vi "realtime_IV_K2182A_K6221_vs_time_PK.vi"() -> ()   [LabVIEW 2016]
uses:
  Labview Drivers/Keithley 622x LV 2009/Keithley 622x LV 2009/Utility/Typedefs/KE622x -- Instrument Type.ctl
  \\home2\scratch/Heng/Vread vs time program/C/Program Files/National Instruments/LabVIEW 2016/instr.lib/Keithley 2182/Keithley 2182.lvlib
  Labview Drivers/Keithley 622x LV 2009/Keithley 622x.lvlib
panel:
  in  "Compliance Voltage (V)":dbl=2.0 format="%#_13g"
  in  "Measurement time (s)":i32=5
  in  "I low (A)":dbl=3.5e-05 format="%#_13g"
  in  "I high (A)":dbl=3.5e-05 format="%#_13g"
  in  "milliseconds to wait":u32=50
  out "Current (A)":dbl=3.5e-05
  out "Voltage, Current vs time":cluster{dbl[], dbl[]}[](graph)=[{[0.09001120005268604, 0.17392860003747046, 0.25689580000471324, 0.34132849995512515, 0.42540299997199327, 0.5330105000175536, 0.616786599974148, 0.7007576000178233, 0.7859523999504745, 0.8734561000019312, 0.9573167000198737, 1.0410527000203729, 1.123987799976021, 1.2319731999887154, 1.3157297000288963, 1.3994928000029176, 1.4842683000024408, 1.567963800043799, 1.6757461000233889, 1.7604933000402525, 1.8453336999518797, 1.9281911000143737, 2.011828999966383, 2.1194837000221014, 2.2033508999738842, 2.288044400047511, 2.3720796999987215, 2.455827399971895, 2.564476400031708, 2.648404399980791, 2.732585599995218, 2.8160608999896795, 2.899973400053568, 3.0093368999660015, 3.0932457000017166, 3.1782505000010133, 3.2620929999975488, 3.34611279994715, 3.4536611000075936, 3.53644890000578, 3.619862799998373, 3.7043840000405908, 3.787445200025104, 3.8964777999790385, 3.9805380000034347, 4.06360069999937, 4.147366099990904, 4.2313554000575095, 4.342785699991509, 4.42666899994947, 4.510417400044389, 4.594143499969505, 4.677875300054438, 4.7866037000203505, 4.868433300056495, 4.950147600029595, 5.03403740003705, 5.116245900047943, 5.225699799950235, 5.309295200044289, 5.392163599957712, 5.475838299957104, 5.559273199993186, 5.668193200021051, 5.751985499984585, 5.8357585000339895, 5.92049509997014, 6.004160400014371, 6.112092899973504, 6.195801900001243, 6.2805609999923036, 6.364234099979512, 6.448114800034091, 6.556113400030881, 6.639614199986681, 6.723240699968301, 6.807079700054601, 6.891112699988298, 6.999815399991348, 7.0835898000514135, 7.167793800006621, 7.251457900041714, 7.335164400050417, 7.442889400059357, 7.525731400004588, 7.609408600023016, 7.693278899998404, 7.776963599957526, 7.887556300032884, 7.971557899960317, 8.055263599962927, 8.139243199955672, 8.221872400026768, 8.376425900030881, 8.460303799947724, 8.544166299980134, 8.627897000056691, 8.711752300034277, 8.819434399949387, 8.902712399954908, 8.985357800032943, 9.069069199962541, 9.152736100018956, 9.261347300023772, 9.344197700032964, 9.4280402000295, 9.512762399972416, 9.59685970004648, 9.707502600038424, 9.789378299959935, 9.873171100043692, 9.956881299964152, 10.040252799983136, 10.149399799993262, 10.232639400055632, 10.315507599967532, 10.39811239996925, 10.483006999944337, 10.589900000020862, 10.673453800030984, 10.75625510001555, 10.838458999991417, 10.921870499965735, 11.030491200042889, 11.112396799959242, 11.195403899997473, 11.279033600003459, 11.36295560002327, 11.47256689995993, 11.556370600010268, 11.639203600003384, 11.723033200018108, 11.806714799953625, 11.915487900027074, 11.997212399961427, 12.081089899991639, 12.164966500014998, 12.248737000045367, 12.357347400044091, 12.439515799982473, 12.523037999984808, 12.606748000020161, 12.69069269997999, 12.798886899952777, 12.882544600055553, 12.966471399995498, 13.050215000053868, 13.134237400023267, 13.245849599945359, 13.329620899981819, 13.413423900026828, 13.497106299968436, 13.580901199951768, 13.688763599959202, 13.772477800026536, 13.856217900058255, 13.939937900053337, 14.02286400005687, 14.131848799996078, 14.215486999950372, 14.299411899992265, 14.383130199974403, 14.466931400005706, 14.574997700052336, 14.658611900056712], [2.01901868e-05, 3.5e-05, 2.02808084e-05, 3.5e-05, 2.01789231e-05, 3.5e-05, 2.01968426e-05, 3.5e-05, 2.0146668e-05, 3.5e-05, 2.02485533e-05, 3.5e-05, 2.02813204e-05, 3.5e-05, 2.01953067e-05, 3.5e-05, 2.02132262e-05, 3.5e-05, 2.0222954e-05, 3.5e-05, 2.00949573e-05, 3.5e-05, 2.01691954e-05, 3.5e-05, 2.02055464e-05, 3.5e-05, 2.01482039e-05, 3.5e-05, 2.02342177e-05, 3.5e-05, 2.01973546e-05, 3.5e-05, 2.02531612e-05, 3.5e-05, 2.01968426e-05, 3.5e-05, 2.02649368e-05, 3.5e-05, 2.01610036e-05, 3.5e-05, 2.02690327e-05, 3.5e-05, 2.01338683e-05, 3.5e-05, 2.02654488e-05, 3.5e-05, 2.01901868e-05, 3.5e-05, 2.02342281e-05, 3.5e-05, 2.02122127e-05, 3.5e-05, 2.01912213e-05, 3.5e-05, 2.01942932e-05, 3.5e-05, 2.02178446e-05, 3.5e-05, 2.01702298e-05, 3.5e-05, 2.01548702e-05, 3.5e-05, 2.02250124e-05, 3.5e-05, 2.01558942e-05, 3.5e-05, 2.02577795e-05, 3.5e-05, 2.01784216e-05, 3.5e-05, 2.02219405e-05, 3.5e-05, 2.02050449e-05, 3.5e-05, 2.02127247e-05, 3.5e-05, 2.02132367e-05, 3.5e-05, 2.0200437e-05, 3.5e-05, 2.01405346e-05, 3.5e-05, 2.01328548e-05, 3.5e-05, 2.02096528e-05, 3.5e-05, 2.01302948e-05, 3.5e-05, 2.01364387e-05, 3.5e-05, 2.01512863e-05, 3.5e-05, 2.02931066e-05, 3.5e-05, 2.01773976e-05, 3.5e-05, 2.02265483e-05, 3.5e-05, 2.01594781e-05, 3.5e-05, 2.02311562e-05, 3.5e-05, 2.0124151e-05, 3.5e-05, 2.02434439e-05, 3.5e-05, 2.01497503e-05, 3.5e-05, 2.02229644e-05, 3.5e-05, 2.01523103e-05, 3.5e-05, 2.01948052e-05, 3.5e-05, 2.0125687e-05, 3.5e-05, 2.0163062e-05, 3.5e-05, 2.01932692e-05, 3.5e-05, 2.00929198e-05, 3.5e-05, 2.02285963e-05, 3.5e-05, 2.01389986e-05, 3.5e-05, 2.02055569e-05, 3.5e-05, 2.01277349e-05, 3.5e-05, 2.01799575e-05, 3.5e-05, 2.01942932e-05, 3.5e-05, 2.01533342e-05, 3.5e-05, 2.0200949e-05, 3.5e-05, 2.01026476e-05, 3.5e-05, 2.01809815e-05, 3.5e-05, 2.00898479e-05, 3.5e-05, 2.01656219e-05, 3.5e-05, 2.01364387e-05, 3.5e-05, 2.01968572e-05, 3.5e-05, 2.008934e-05, 3.5e-05, 2.01226191e-05, 3.5e-05, 2.01144273e-05, 3.5e-05, 2.01077715e-05, 3.5e-05, 2.01128914e-05, 3.5e-05, 2.01057235e-05, 3.5e-05, 2.01799616e-05, 3.5e-05, 2.01748418e-05]}, {[0.09001120005268604, 0.17392860003747046, 0.25689580000471324, 0.34132849995512515, 0.42540299997199327, 0.5330105000175536, 0.616786599974148, 0.7007576000178233, 0.7859523999504745, 0.8734561000019312, 0.9573167000198737, 1.0410527000203729, 1.123987799976021, 1.2319731999887154, 1.3157297000288963, 1.3994928000029176, 1.4842683000024408, 1.567963800043799, 1.6757461000233889, 1.7604933000402525, 1.8453336999518797, 1.9281911000143737, 2.011828999966383, 2.1194837000221014, 2.2033508999738842, 2.288044400047511, 2.3720796999987215, 2.455827399971895, 2.564476400031708, 2.648404399980791, 2.732585599995218, 2.8160608999896795, 2.899973400053568, 3.0093368999660015, 3.0932457000017166, 3.1782505000010133, 3.2620929999975488, 3.34611279994715, 3.4536611000075936, 3.53644890000578, 3.619862799998373, 3.7043840000405908, 3.787445200025104, 3.8964777999790385, 3.9805380000034347, 4.06360069999937, 4.147366099990904, 4.2313554000575095, 4.342785699991509, 4.42666899994947, 4.510417400044389, 4.594143499969505, 4.677875300054438, 4.7866037000203505, 4.868433300056495, 4.950147600029595, 5.03403740003705, 5.116245900047943, 5.225699799950235, 5.309295200044289, 5.392163599957712, 5.475838299957104, 5.559273199993186, 5.668193200021051, 5.751985499984585, 5.8357585000339895, 5.92049509997014, 6.004160400014371, 6.112092899973504, 6.195801900001243, 6.2805609999923036, 6.364234099979512, 6.448114800034091, 6.556113400030881, 6.639614199986681, 6.723240699968301, 6.807079700054601, 6.891112699988298, 6.999815399991348, 7.0835898000514135, 7.167793800006621, 7.251457900041714, 7.335164400050417, 7.442889400059357, 7.525731400004588, 7.609408600023016, 7.693278899998404, 7.776963599957526, 7.887556300032884, 7.971557899960317, 8.055263599962927, 8.139243199955672, 8.221872400026768, 8.376425900030881, 8.460303799947724, 8.544166299980134, 8.627897000056691, 8.711752300034277, 8.819434399949387, 8.902712399954908, 8.985357800032943, 9.069069199962541, 9.152736100018956, 9.261347300023772, 9.344197700032964, 9.4280402000295, 9.512762399972416, 9.59685970004648, 9.707502600038424, 9.789378299959935, 9.873171100043692, 9.956881299964152, 10.040252799983136, 10.149399799993262, 10.232639400055632, 10.315507599967532, 10.39811239996925, 10.483006999944337, 10.589900000020862, 10.673453800030984, 10.75625510001555, 10.838458999991417, 10.921870499965735, 11.030491200042889, 11.112396799959242, 11.195403899997473, 11.279033600003459, 11.36295560002327, 11.47256689995993, 11.556370600010268, 11.639203600003384, 11.723033200018108, 11.806714799953625, 11.915487900027074, 11.997212399961427, 12.081089899991639, 12.164966500014998, 12.248737000045367, 12.357347400044091, 12.439515799982473, 12.523037999984808, 12.606748000020161, 12.69069269997999, 12.798886899952777, 12.882544600055553, 12.966471399995498, 13.050215000053868, 13.134237400023267, 13.245849599945359, 13.329620899981819, 13.413423900026828, 13.497106299968436, 13.580901199951768, 13.688763599959202, 13.772477800026536, 13.856217900058255, 13.939937900053337, 14.02286400005687, 14.131848799996078, 14.215486999950372, 14.299411899992265, 14.383130199974403, 14.466931400005706, 14.574997700052336, 14.658611900056712], [3.5e-05, 2.01727793e-05, 3.5e-05, 2.02393375e-05, 3.5e-05, 2.02132262e-05, 3.5e-05, 2.02552091e-05, 3.5e-05, 2.02024745e-05, 3.5e-05, 2.02255139e-05, 3.5e-05, 2.01502519e-05, 3.5e-05, 2.02475293e-05, 3.5e-05, 2.01220926e-05, 3.5e-05, 2.02347296e-05, 3.5e-05, 2.01615156e-05, 3.5e-05, 2.02552091e-05, 3.5e-05, 2.02086183e-05, 3.5e-05, 2.01953067e-05, 3.5e-05, 2.01226046e-05, 3.5e-05, 2.02695447e-05, 3.5e-05, 2.01569077e-05, 3.5e-05, 2.02188581e-05, 3.5e-05, 2.0183019e-05, 3.5e-05, 2.01947947e-05, 3.5e-05, 2.01748272e-05, 3.5e-05, 2.02101543e-05, 3.5e-05, 2.01666354e-05, 3.5e-05, 2.01558942e-05, 3.5e-05, 2.01861014e-05, 3.5e-05, 2.02070928e-05, 3.5e-05, 2.01820055e-05, 3.5e-05, 2.01779096e-05, 3.5e-05, 2.02280843e-05, 3.5e-05, 2.01661339e-05, 3.5e-05, 2.02183566e-05, 3.5e-05, 2.01912213e-05, 3.5e-05, 2.01809815e-05, 3.5e-05, 2.02296203e-05, 3.5e-05, 2.01517983e-05, 3.5e-05, 2.02613634e-05, 3.5e-05, 2.02495877e-05, 3.5e-05, 2.0240372e-05, 3.5e-05, 2.01364387e-05, 3.5e-05, 2.02070928e-05, 3.5e-05, 2.02035089e-05, 3.5e-05, 2.02229644e-05, 3.5e-05, 2.01799575e-05, 3.5e-05, 2.01922452e-05, 3.5e-05, 2.02035089e-05, 3.5e-05, 2.02157966e-05, 3.5e-05, 2.01804695e-05, 3.5e-05, 2.01973651e-05, 3.5e-05, 2.01072554e-05, 3.5e-05, 2.02117007e-05, 3.5e-05, 2.02137487e-05, 3.5e-05, 2.02050449e-05, 3.5e-05, 2.02367881e-05, 3.5e-05, 2.01881493e-05, 3.5e-05, 2.0199413e-05, 3.5e-05, 2.01948052e-05, 3.5e-05, 2.01692058e-05, 3.5e-05, 2.01768856e-05, 3.5e-05, 2.0238324e-05, 3.5e-05, 2.01507743e-05, 3.5e-05, 2.01425825e-05, 3.5e-05, 2.01712538e-05, 3.5e-05, 2.01471904e-05, 3.5e-05, 2.01814935e-05, 3.5e-05, 2.01400226e-05, 3.5e-05, 2.02183566e-05, 3.5e-05, 2.01441185e-05, 3.5e-05, 2.02219405e-05, 3.5e-05, 2.01748377e-05, 3.5e-05, 2.01477024e-05, 3.5e-05, 2.01912213e-05, 3.5e-05, 2.01420705e-05, 3.5e-05, 2.0201973e-05, 3.5e-05, 2.00918999e-05, 3.5e-05, 2.0203001e-05, 3.5e-05, 2.0087804e-05, 3.5e-05, 2.01850815e-05, 3.5e-05, 2.01046996e-05, 3.5e-05, 2.0128763e-05, 3.5e-05, 2.00688605e-05, 3.5e-05, 2.01789377e-05, 3.5e-05, 2.00791002e-05, 3.5e-05]}]
  in  "Instrument Type":T1=enum."KE6221"
  in  "K6221":refnum<visa-resource-name>="GPIB0::12::INSTR"
  out "Time(s)":dbl=14.742446399992332 format="%#_13g"
  in  "?":bool
  out "Voltage (V)":dbl=2.01748418e-05
  in  "Folder":path=path "D:/Banabir/Second round/11-04-2021"
  out "data":dbl[](array[numeric])=[14.658611900056712, 3.5e-05, 2.01748418e-05]
  in  "Nanovoltmeter K2182A VISA (Device 1)":refnum<visa-resource-name>="GPIB0::4::INSTR"
  in  "file name":string="test6"
  out "File path":path=path "D:/Banabir/Second round/11-04-2021/test6.dat"
  # ".dat"
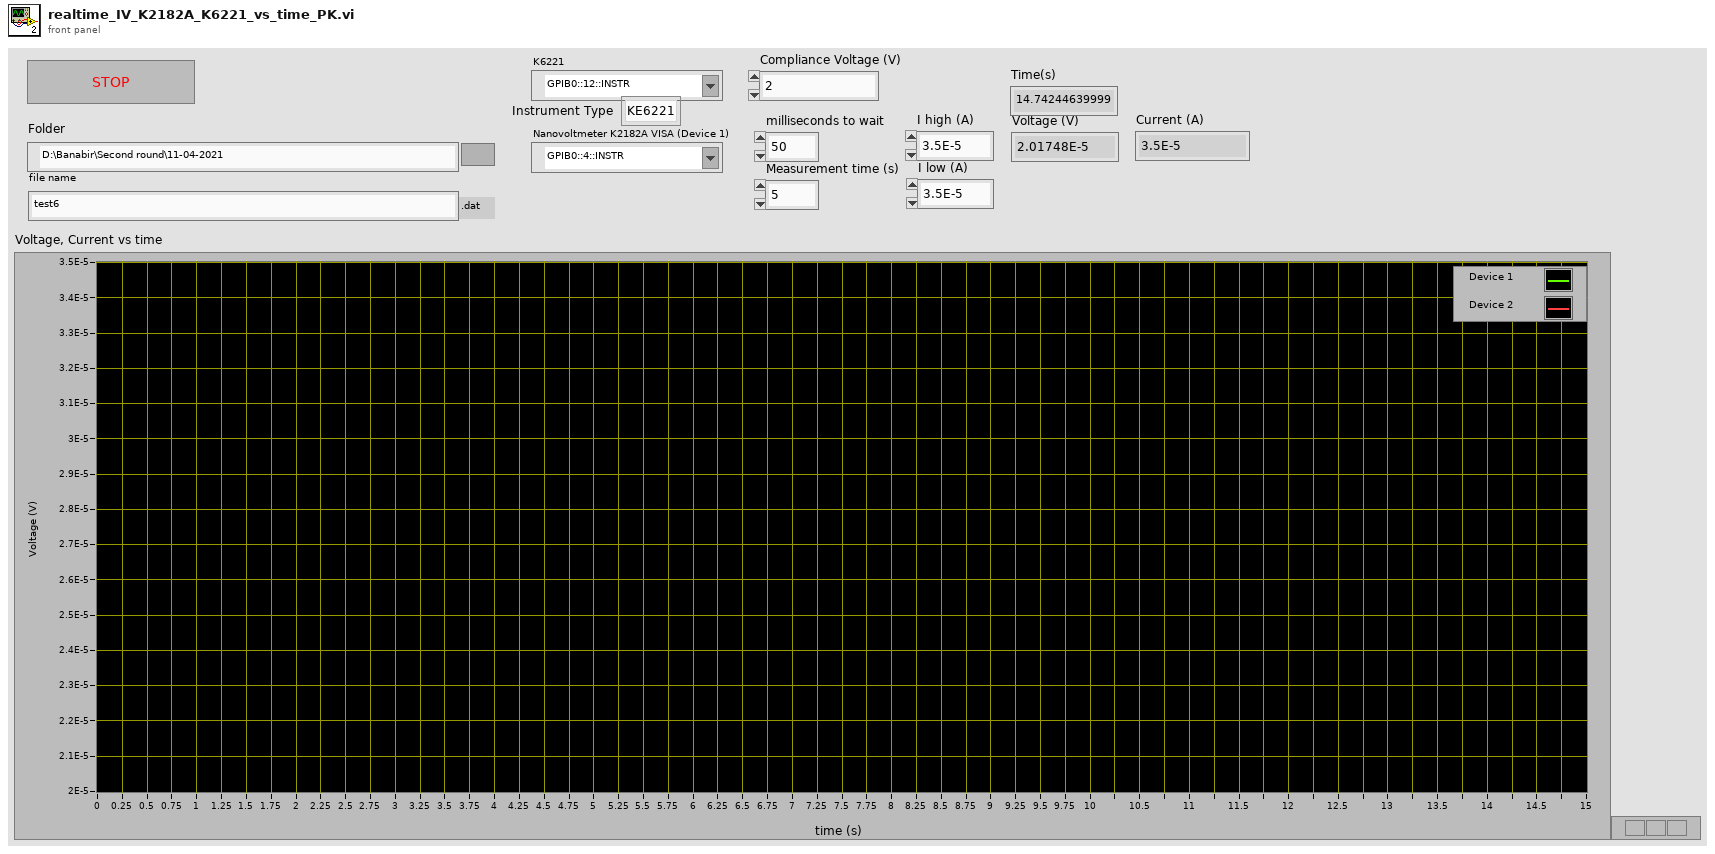
[diagram p1: front panel]
types:
  T1 = typedef "Keithley 622x.lvlib/KE622x -- Instrument Type.ctl" = enum16{"KE6220", "KE6221"}
  T2 = enum16{"open", "replace", "create", "open or create", "replace or create", "replace or create with confirmation"}
  T3 = typedef "Keithley 622x.lvlib/KE622x -- Current Level.ctl" = dbl
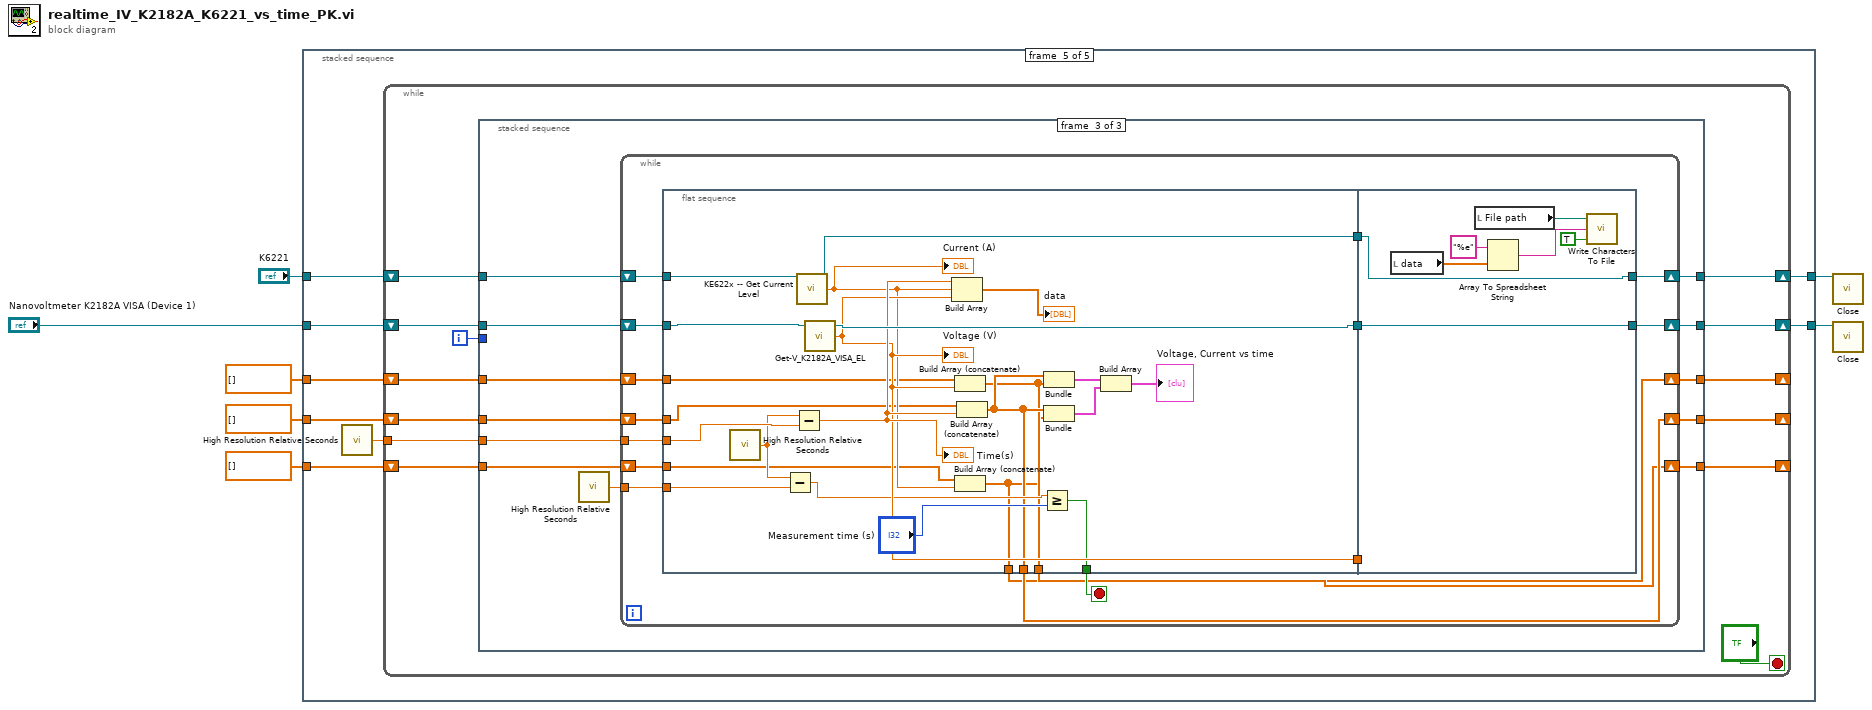
[diagram p0: block diagram]
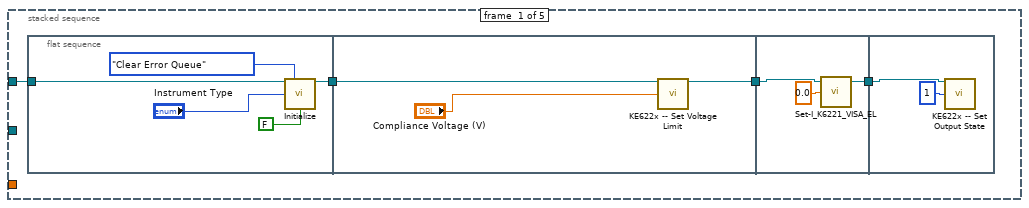
[diagram p2: hidden frame]
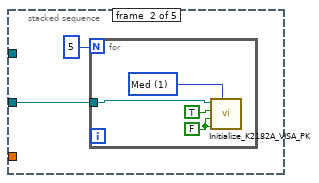
[diagram p3: hidden frame]
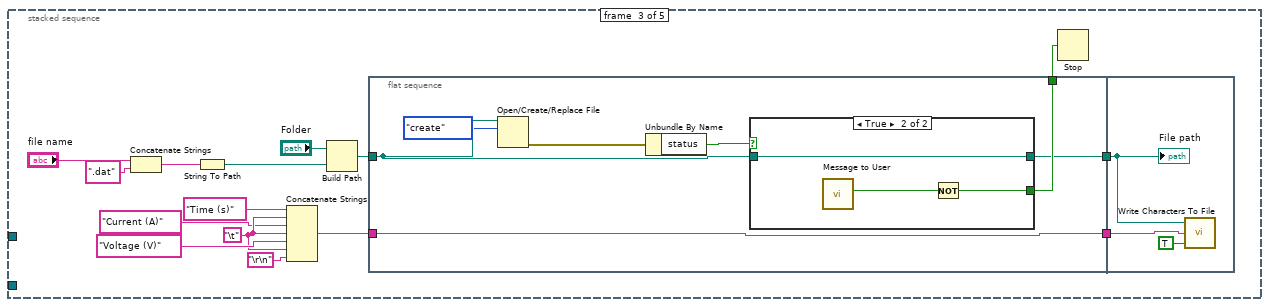
[diagram p4: hidden frame]
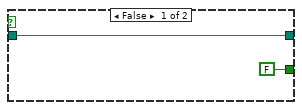
[diagram p5: hidden frame]
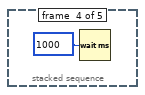
[diagram p6: hidden frame]
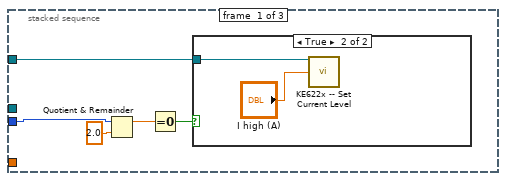
[diagram p7: hidden frame]
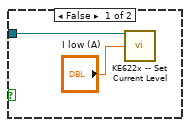
[diagram p8: hidden frame]
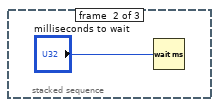
[diagram p9: hidden frame]
diagram:
  n1 = stacked-sequence {
    tunnel: "Nanovoltmeter K2182A VISA (Device 1)" -> [_ w25 _ _ w69]
    tunnel: [_ _ _ _ w67] -> w6
    tunnel: "K6221" -> [w11 _ _ _ w66]
    tunnel: [_ _ _ _ w65] -> w4
    tunnel: dbl[] [] -> [_ _ _ _ w64]
    tunnel: dbl[] [] -> [_ _ _ _ w63]
    tunnel: dbl[] [] -> [_ _ _ _ w62]
    frame #0 {
      n2 = flat-sequence {
        tunnel: w11 -> [w16]
        tunnel: [w15] -> w9
        tunnel: w9 -> [w18]
        tunnel: [w19] -> w8
        tunnel: w8 -> [w21]
        tunnel: [w20] -> w10
        tunnel: w10 -> [w23]
        frame #0 {
          n3 = call "Initialize.vi"("VISA resource name"=w16, "Error Queue Option"=enum16{"Clear Error Queue", "Error Query"}."Clear Error Queue", "Instrument Type"="Instrument Type", "Reset? (T)"=FALSE) -> ("VISA resource name out"=w15:refnum<visa-resource-name>)  [unwired: 10 in, 1 out]
        }
        frame #1 {
          n4 = call "KE622x -- Set Voltage Limit.vi"("Resource In"=w18, "Voltage Limit (V)"="Compliance Voltage (V)") -> ("Resource Out (dupl)"=w19:refnum<visa-resource-name>)  [unwired: 12 in, 1 out]
        }
        frame #2 {
          n5 = call "Set-I_K6221_VISA_EL.vi"("Set I (A)"=0.0, "K6221 VISA"=w21) -> ("K6221 VISA out"=w20:refnum<visa-resource-name>)  [unwired: 2 in, 1 out]
        }
        frame #3 {
          n6 = call "KE622x -- Set Output State.vi"("Resource In"=w23, "Output State"=1) -> ()  [unwired: 12 in, 2 out]
        }
      }
    }
    frame #1 {
      n7 = for {
        N: 5 ("Numeric") -> [_]
        tunnel: w25 -> [w27]
        w29 = u16 1 items=["Slow", "Med", "Fast"] ("Rate (NPLC)")
        w30 = FALSE ("Auto range?")
        n8 = call "Initialize_K2182A_VISA_PK.vi"("VISA address"=w27, "Auto range?"=TRUE, "Analog LPass\nFilter?"=w30, "DC\nFilter?"=w30, "Rate (NPLC)"=w29) -> ()  [unwired: 2 in]
      }
    }
    frame #2 {
      w32 = "\t"
      n9 = Concatenate Strings("file name", ".dat" ("string")) -> (w42:string)
      n10 = String To Path(string=w42) -> (path=w35:path)
      n11 = Concatenate Strings("Time (s)" ("string"), w32, "Current (A)", w32, "Voltage (V)" ("string"), w32, "\r\n") -> (w43:string)
      n12 = Build Path(base path="Folder", name or relative path=w35) -> (appended path=w34:path)
      n13 = flat-sequence {
        tunnel: w34 -> [w49]
        tunnel: w43 -> [w52]
        tunnel: [w52] -> w45
        tunnel: [w51] -> w40
        tunnel: [w50] -> w44
        tunnel: w45 -> [w59]
        tunnel: w44 -> [w58]
        frame #0 {
          n14 = Open/Create/Replace File(file path (use dialog)=w49, operation (0:open)=T2."create") -> (error out=w48:errorcluster)  [unwired: 4 in, 2 out]
          n15 = Unbundle By Name(w48) -> ("status"=w46:bool)
          n16 = case shown="True" w46 {
            tunnel: [FALSE ("Yes") w56] -> w51
            tunnel: [w53 w55] -> w50
            tunnel: w49 -> [w53 w55]
            frame False {
            }
            frame True {
              n17 = call "Message to User"() -> ("Yes"=w57:bool)  [unwired: 10 in, 1 out]
              n18 = Not(x=w57) -> (.not. x?=w56:bool)
            }
          }
        }
        frame #1 {
          n19 = call <vilib>:"Write Characters To File.vi"("append to file? (new file:F)"=TRUE, "character string"=w59, "file path (dialog if empty)"=w58) -> ()  [unwired: 2 in, 1 out]
          "File path" <- w58
        }
      }
      n20 = Stop(stop? (T)=w40) -> ()
    }
    frame #3 {
      n21 = Wait (ms)(milliseconds to wait=u32 1000) -> ()  [unwired: 1 out]
    }
    frame #4 {
      n22 = call <vilib>:"High Resolution Relative Seconds.vi"() -> ("relative seconds"=w68:dbl)
      n23 = while {
        shift-right: [w80] -> w67
        shift-left: w69 -> [w82]
        tunnel: w68 -> [w79]
        shift-right: [w74] -> w65
        shift-left: w66 -> [w75]
        shift-right: [w71] -> _
        shift-left: w62 -> [w78]
        shift-right: [w70] -> _
        shift-left: w64 -> [w77]
        shift-right: [w72] -> _
        shift-left: w63 -> [w76]
        i -> [w73]
        stop <- "?" stop-if-true
        n24 = stacked-sequence {
          tunnel: w82 -> [_ _ w104]
          tunnel: [_ _ w103] -> w80
          tunnel: w79 -> [_ _ w102]
          tunnel: w75 -> [w83 _ w101]
          tunnel: w78 -> [_ _ w99]
          tunnel: w77 -> [_ _ w97]
          tunnel: w76 -> [_ _ w98]
          tunnel: [_ _ w100] -> w74
          tunnel: w73 -> [w87 _ _]
          tunnel: [_ _ w95] -> w72
          tunnel: [_ _ w94] -> w71
          tunnel: [_ _ w93] -> w70
          frame #0 {
            n25 = Quotient & Remainder(x=w87, y=2.0) -> (x-y*floor(x/y)=w85:dbl)  [unwired: 1 out]
            n26 = Equal To 0?(x=w85) -> (x = 0?=w84:bool)
            n27 = case shown="True" w84 {
              tunnel: w83 -> [w88 w90]
              frame False {
                n28 = call "KE622x -- Set Current Level.vi"("Resource In"=w88, "Current Level (A) In"="I low (A)") -> ()  [unwired: 11 in, 3 out]
              }
              frame True {
                n29 = call "KE622x -- Set Current Level.vi"("Resource In"=w90, "Current Level (A) In"="I high (A)") -> ()  [unwired: 11 in, 3 out]
              }
            }
          }
          frame #1 {
            n30 = Wait (ms)(milliseconds to wait="milliseconds to wait") -> ()  [unwired: 1 out]
          }
          frame #2 {
            n31 = call <vilib>:"High Resolution Relative Seconds.vi"() -> ("relative seconds"=w96:dbl)
            n32 = while {
              shift-right: [w119] -> w103
              shift-left: w104 -> [w120]
              shift-right: [w116] -> w100
              shift-left: w101 -> [w117]
              tunnel: w96 -> [w112]
              shift-right: [w106] -> w95
              shift-left: w98 -> [w114]
              shift-right: [w105] -> w93
              shift-left: w97 -> [w113]
              shift-right: [w107] -> w94
              shift-left: w99 -> [w115]
              tunnel: w102 -> [w118]
              stop <- w111 stop-if-true
              n33 = flat-sequence {
                tunnel: w120 -> [w142]
                tunnel: w118 -> [w140]
                tunnel: w117 -> [w137]
                tunnel: w115 -> [w125]
                tunnel: w114 -> [w127]
                tunnel: w113 -> [w126]
                tunnel: w112 -> [w132]
                tunnel: [w128] -> w111
                tunnel: [w141] -> w110
                tunnel: [w138] -> w109
                tunnel: [w136] -> w108
                tunnel: [w123] -> w107
                tunnel: [w122] -> w106
                tunnel: [w121] -> w105
                tunnel: [w149] -> w116
                tunnel: [w150] -> w119
                tunnel: w110 -> [w150]
                tunnel: w109 -> [_]
                tunnel: w108 -> [w149]
                frame #0 {
                  n34 = call <vilib>:"High Resolution Relative Seconds.vi"() -> ("relative seconds"=w131:dbl)
                  n35 = Subtract(x=w131, y=w132) -> (x-y=w130:dbl)
                  n36 = Subtract(x=w131, y=w140) -> (x-y=w139:dbl)
                  "Time(s)" <- w139
                  n37 = call "KE622x -- Get Current Level.vi"("Resource In"=w137) -> ("Resource Out (dupl)"=w136:refnum<visa-resource-name>, "Current Level (A)"=w135:T3)  [unwired: 12 in, 1 out]
                  "Current (A)" <- w135
                  n38 = call "Get-V_K2182A_VISA_EL.vi"("VISA K2182A"=w142) -> ("V (V)"=w138:dbl, "VISA K2182A"=w141:refnum<visa-resource-name>)  [unwired: 2 in, 1 out]
                  "Voltage (V)" <- w138
                  n39 = Build Array(w139, w135, w138) -> (→"data":T3[])
                  n40 = Build Array (concatenate)(w126, w138) -> (w122:T3[])
                  n41 = Build Array (concatenate)(w127, w135) -> (w121:T3[])
                  n42 = Build Array (concatenate)(w125, w139) -> (w123:dbl[])
                  n43 = Greater Or Equal?(x=w130, y="Measurement time (s)") -> (x >= y?=w128:bool)
                  n44 = Bundle(w123, w122) -> (w134:cluster{dbl[], T3[]})  [unwired: 1 in]
                  n45 = Bundle(w123, w121) -> (w124:cluster{dbl[], T3[]})  [unwired: 1 in]
                  n46 = Build Array(w134, w124) -> (→"Voltage, Current vs time":cluster{dbl[], T3[]}[])
                }
                frame #1 {
                  n47 = local read "data"() -> (w144:dbl[])
                  n48 = local read "File path"() -> (w146:path)
                  n49 = Array To Spreadsheet String(array=w144, 3:"%e" ("format string")) -> (spreadsheet string=w147:string)  [unwired: 1 in]
                  n50 = call <vilib>:"Write Characters To File.vi"("append to file? (new file:F)"=TRUE, "character string"=w147, "file path (dialog if empty)"=w146) -> ()  [unwired: 2 in, 1 out]
                }
              }
            }
          }
        }
      }
    }
  }
  n51 = call "Close.vi"("VISA resource name"=w4) -> ()  [unwired: 14 in, 1 out]
  n52 = call "Close.vi"("VISA resource name"=w6) -> ()  [unwired: 10 in, 1 out]
